vi "Set Initialize Hot And Cold Source Unit.vi"(8 "error in (no error)":errorcluster, 10 "Initialize Hot And Cold Source Unit":bool, 11 "Abstract Initialize Hot And Cold Source Unit Msg in":refnum<class "Abstract Initialize Hot And Cold Source Unit Msg.lvclass">) -> (0 "error out":errorcluster, 3 "Abstract Initialize Hot And Cold Source Unit Msg out":refnum<class "Abstract Initialize Hot And Cold Source Unit Msg.lvclass">)   [LabVIEW 2013, in "Hot And Cold Source Unit Model.lvlib" / "Abstract Initialize Hot And Cold Source Unit Msg.lvclass"]
uses:
  Abstract Initialize Hot And Cold Source Unit Msg.lvclass
  Abstract Initialize Hot And Cold Source Unit Msg.lvclass/Abstract Initialize Hot And Cold Source Unit Msg.ctl
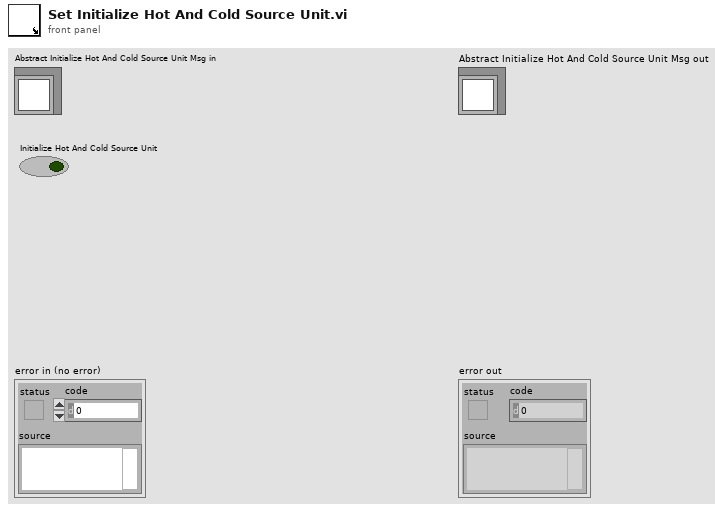
[diagram p1: front panel]
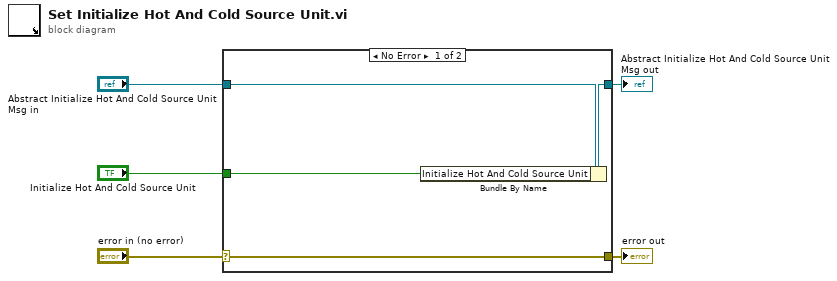
[diagram p0: block diagram]
diagram:
  n1 = case shown="No Error" "error in (no error)" {
    selector: "error in (no error)" -> [w9 w10]
    tunnel: [w9 w10] -> w4
    tunnel: [w7 w11] -> w2
    tunnel: "Abstract Initialize Hot And Cold Source Unit Msg in" -> [w8 w11]
    tunnel: "Initialize Hot And Cold Source Unit" -> [w6 _]
    frame No Error {
      n2 = Bundle By Name(cluster=w8, "Initialize Hot And Cold Source Unit"=w6) -> (w7:refnum<class "Abstract Initialize Hot And Cold Source Unit Msg.lvclass">)
    }
    frame Error {
    }
  }
  "error out" <- w4
  "Abstract Initialize Hot And Cold Source Unit Msg out" <- w2
